vi "Update Reversi Project.vi"() -> ()   [LabVIEW 2020]
uses:
  dev/Version.ctl
  dev/Updater State.ctl
  c5f3ca88-f85c-4b21-a54c-2e2b82621a56.vi
  fab92dee-f5cc-474f-8dc6-a01214f8643b.vi
  <vilib>/Comparison/Equal/Equal Functor/Equal Functor.lvclass
panel:
  out "Project":refnum<vi>
  out "Template Vers Str":string
  out "Project Vers Str":string
  out "Template Version":T1
  out "Project Version":T1
  out "NonOOP Template":path
  out "Progress":u16(slide) scale=0.0..100.0
  out "Status":string
  out "Players":path[](array[path])
  out "OOP Template":path
  out "Engine Folder":path
  out "Project Path":path
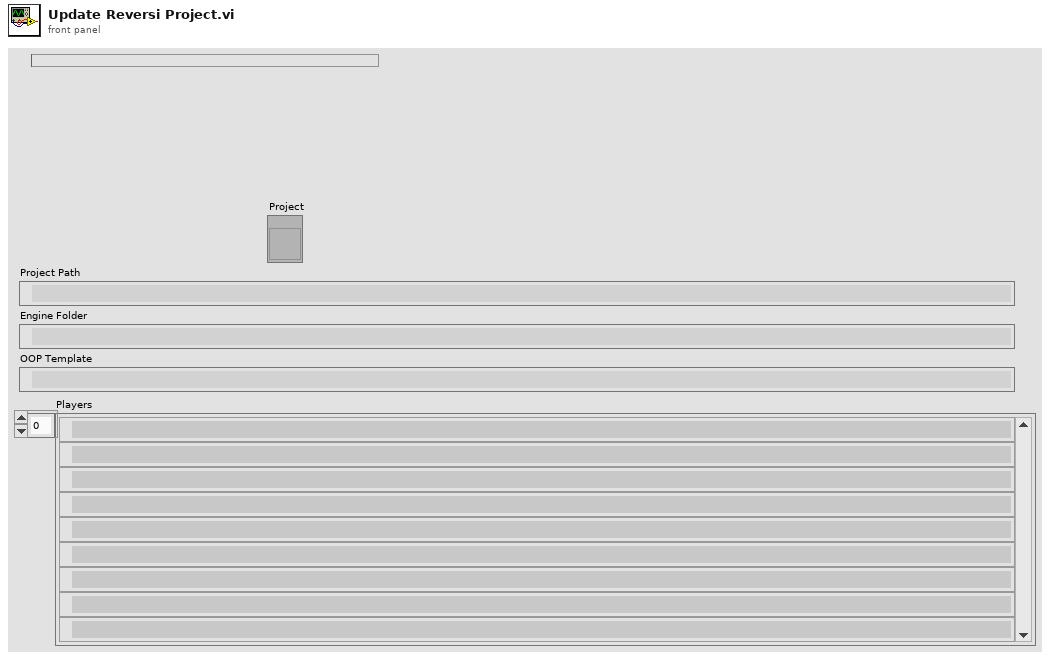
[diagram p1: front panel]
types:
  T1 = typedef "Version.ctl" = cluster{"Major":u16, "Minor":u16, "Fix":u16, "Build":u16}
  T2 = typedef "Updater State.ctl" = enum16{"Get References", "Check Versions", "Confirm", "Close Project", "Copy Engine", "Copy Players", "Open Project", "Version Scripting", "Close"}
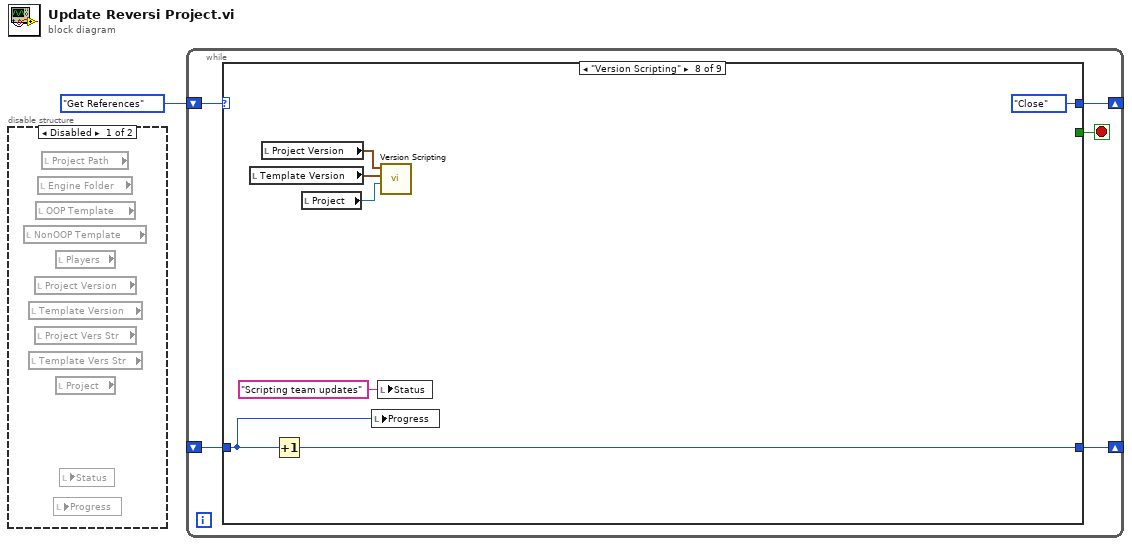
[diagram p0: block diagram]
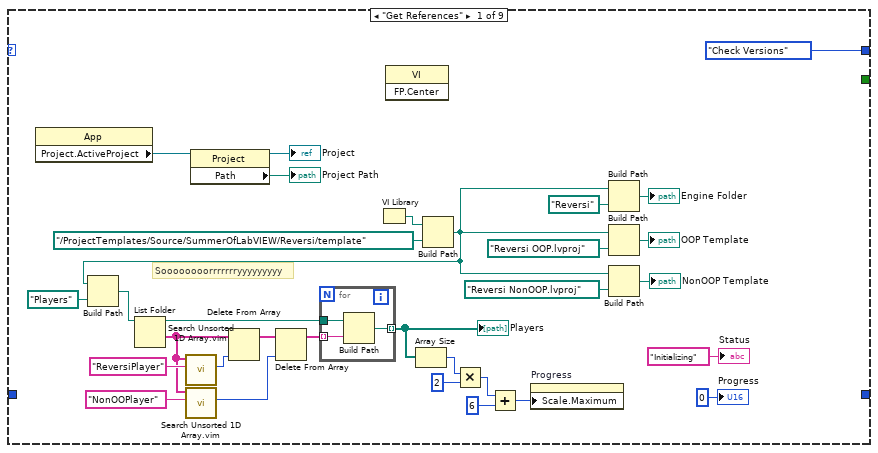
[diagram p3: hidden frame]
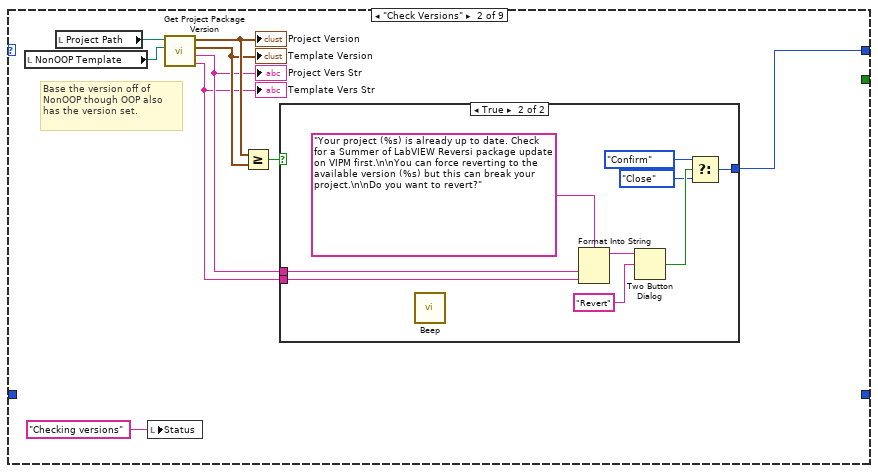
[diagram p4: hidden frame]
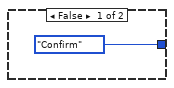
[diagram p5: hidden frame]
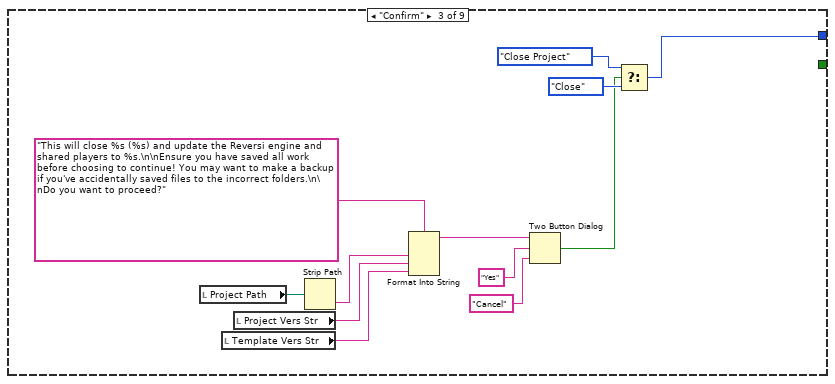
[diagram p6: hidden frame]
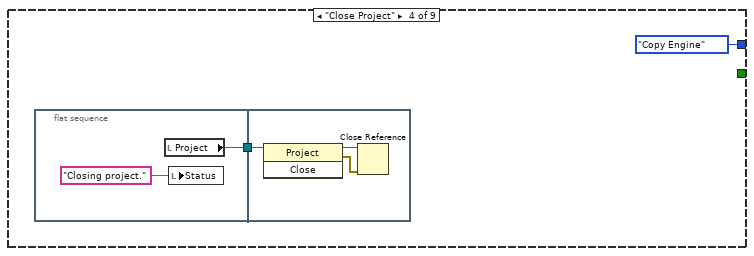
[diagram p7: hidden frame]
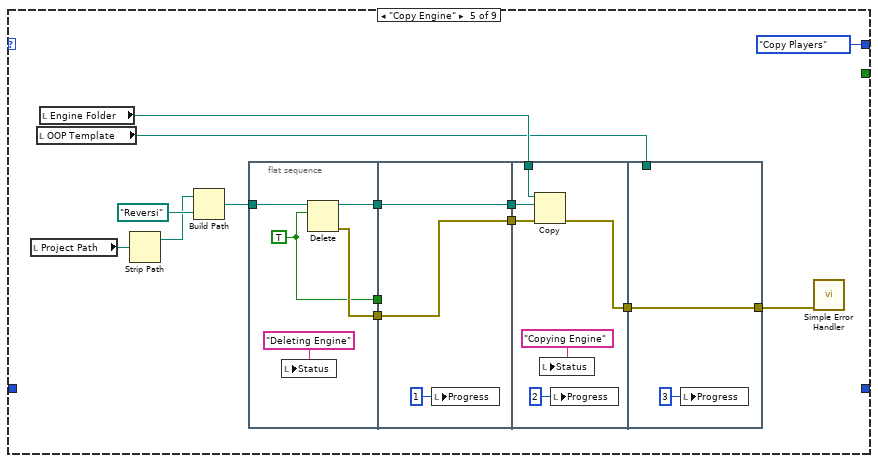
[diagram p8: hidden frame]
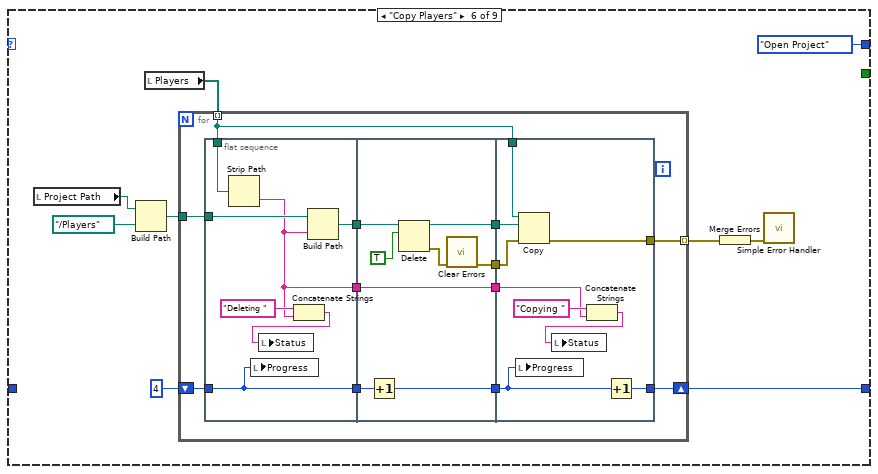
[diagram p9: hidden frame]
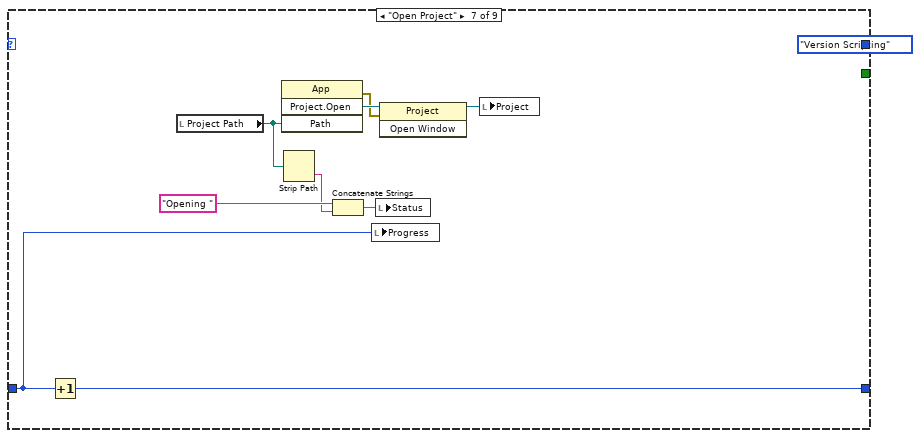
[diagram p10: hidden frame]
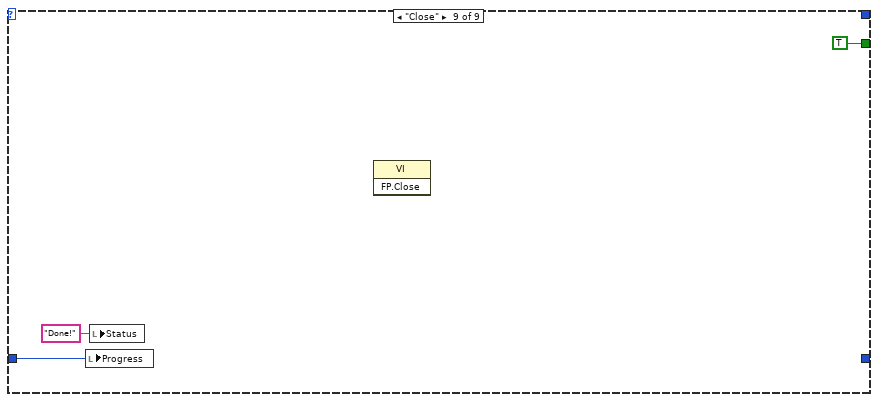
[diagram p11: hidden frame]
diagram:
  n1 = disable-structure shown="Disabled" {
    frame Disabled {
      n2 = local read "NonOOP Template"() -> ()  [unwired: 1 out]
      n3 = local read "Template Version"() -> ()  [unwired: 1 out]
      n4 = local read "Template Vers Str"() -> ()  [unwired: 1 out]
      n5 = local read "Project Version"() -> ()  [unwired: 1 out]
      n6 = local read "Project Vers Str"() -> ()  [unwired: 1 out]
      n7 = local read "OOP Template"() -> ()  [unwired: 1 out]
      n8 = local read "Engine Folder"() -> ()  [unwired: 1 out]
      n9 = local read "Project Path"() -> ()  [unwired: 1 out]
      n10 = local read "Progress"() -> ()  [unwired: 1 in]
      n11 = local read "Players"() -> ()  [unwired: 1 out]
      n12 = local read "Project"() -> ()  [unwired: 1 out]
      n13 = local read "Status"() -> ()  [unwired: 1 in]
    }
    frame Enabled {
    }
  }
  n14 = while {
    shift-right: [w5] -> _
    shift-left: Updater_State."Get References" -> [w6]
    shift-right: [w3] -> _
    shift-left: _ -> [w2]
    stop <- w4 stop-if-true
    n15 = case shown="\"Version Scripting\"" w6 {
      tunnel: [Updater_State."Check Versions" ("f") w43 w66 Updater_State."Copy Engine" ("f") Updater_State."Copy Players" ("f") Updater_State."Open Project" ("f") Updater_State."Version Scripting" ("f") Updater_State."Close" ("f") _] -> w5
      tunnel: [_ _ _ _ _ _ _ _ TRUE] -> w4
      tunnel: [_ _ _ _ _ w109 w155 w164 _] -> w3
      tunnel: w2 -> [_ _ _ _ _ _ w156 w165 w172]
      frame "Get References" {
        # "Soooooooorrrrrrryyyyyyyyy"
        n16 = property class="App"() -> ("Project.ActiveProject"=w15:refnum<vi>)  [unwired: 2 in, 2 out]
        n17 = property class="Project"(reference=w15) -> (reference out=→"Project":refnum<vi>, "Path"=→"Project Path":path)  [unwired: 1 in, 1 out]
        n18 = VI Library() -> (path=w35:path)
        n19 = invoke class="VI" method="FP.Center"() -> ()  [unwired: 3 in, 3 out]
        n20 = Build Path(base path=w35, name or relative path=path "../ProjectTemplates/Source/SummerOfLabVIEW/Reversi/template") -> (appended path=w14:path)
        n21 = Build Path(base path=w14, name or relative path=path "Players") -> (appended path=w28:path)
        n22 = List Folder(path=w28) -> (path out=w25:path, folder names=w10:string[])  [unwired: 3 in, 2 out]
        n23 = call "Search Unsorted 1D Array.vim"("element"="ReversiPlayer", "unsorted 1D array"=w10) -> ("index of element"=w26:i32)  [unwired: 9 in]
        n24 = call "Search Unsorted 1D Array.vim"("element"="NonOOPlayer", "unsorted 1D array"=w10) -> ("index of element"=w8:i32)  [unwired: 9 in]
        n25 = Delete From Array(array=w10, index=w26) -> (array with subset deleted=w9:string[])  [unwired: 1 in, 1 out]
        n26 = Delete From Array(array=w9, index=w8) -> (array with subset deleted=w7:string[])  [unwired: 1 in, 1 out]
        n27 = for {
          tunnel: w7 -> [w39] mode=indexing
          tunnel: w25 -> [w40]
          tunnel: [w38] -> w23 mode=indexing
          n28 = Build Path(base path=w40, name or relative path=w39) -> (appended path=w38:path)
        }
        "Players" <- w23
        n29 = Array Size(array=w23) -> (size(s)=w22:i32)
        n30 = Multiply(x=w22, y=2) -> (x*y=w20:i32)
        n31 = Add(x=w20, y=6) -> (x+y=w18:i32)
        n32 = property on="Progress" class="Slide (strict)"("Scale.Maximum"=w18) -> ()  [unwired: 2 in, 2 out]
        n33 = Build Path(base path=w14, name or relative path=path "Reversi") -> (appended path=→"Engine Folder":path)
        n34 = Build Path(base path=w14, name or relative path=path "Reversi OOP.lvproj") -> (appended path=→"OOP Template":path)
        n35 = Build Path(base path=w14, name or relative path=path "Reversi NonOOP.lvproj") -> (appended path=→"NonOOP Template":path)
        "Status" <- "Initializing" ("Status")
        "Progress" <- u16 0 ("Progress")
      }
      frame "Check Versions" {
        # "Base the version off of NonOOP though OOP also has the version set."
        n36 = local read "NonOOP Template"() -> (w47:path)
        n37 = local read "Project Path"() -> (w49:path)
        n38 = local write "Status"("Checking versions" ("Status")) -> ()
        n39 = call "Get Project Package Version.vi"("Template Project"=w47, "Project Path"=w49) -> ("Template Vers Str"=w41:string, "Project Vers Str"=w42:string, "Template Version"=w45:T1, "Project Version"=w46:T1)  [unwired: 6 in]
        "Project Version" <- w46
        "Template Version" <- w45
        "Project Vers Str" <- w42
        "Template Vers Str" <- w41
        n40 = Greater Or Equal?(x=w46, y=w45) -> (x >= y?=w44:bool)
        n41 = case shown="True" w44 {
          tunnel: [Updater_State."Confirm" ("f") w51] -> w43
          tunnel: w42 -> [_ w58]
          tunnel: w41 -> [_ w57]
          frame False {
          }
          frame True {
            n42 = call <vilib>:"Beep.vi"() -> ()  [unwired: 12 in]
            n43 = Format Into String(format string="Your project (%s) is already up to date. Check for a Summer of LabVIEW Reversi package update on VIPM first.\n\nYou can force reverting to the available version (%s) but this can break your project.\n\nDo you want to revert?" ("message"), w58, w57) -> (resulting string=w56:string)  [unwired: 2 in, 1 out]
            n44 = Two Button Dialog(message=w56, 2:"Revert" ("T button name (\"OK\")")) -> (T button?=w54:bool)  [unwired: 1 in]
            n45 = Select(t=Updater_State."Confirm" ("f"), s=w54, f=Updater_State."Close") -> (s? t:f=w51:T2)
          }
        }
      }
      frame "Confirm" {
        n46 = local read "Project Path"() -> (w64:path)
        n47 = local read "Template Vers Str"() -> (w60:string)
        n48 = local read "Project Vers Str"() -> (w61:string)
        n49 = Strip Path(path=w64) -> (name=w63:string)  [unwired: 1 out]
        n50 = Format Into String(format string="This will close %s (%s) and update the Reversi engine and shared players to %s.\n\nEnsure you have saved all work before choosing to continue! You may want to make a backup if you've accidentally saved files to the incorrect folders.\n\nDo you want to proceed?" ("message"), w63, w61, w60) -> (resulting string=w62:string)  [unwired: 2 in, 1 out]
        n51 = Two Button Dialog(message=w62, 1:"Cancel" ("F button name (\"Cancel\")"), 2:"Yes" ("T button name (\"OK\")")) -> (T button?=w67:bool)
        n52 = Select(t=Updater_State."Close Project", s=w67, f=Updater_State."Close") -> (s? t:f=w66:T2)
      }
      frame "Close Project" {
        n53 = flat-sequence {
          tunnel: [w74] -> w72
          tunnel: w72 -> [w76]
          frame #0 {
            n54 = local read "Project"() -> (w74:refnum<vi>)
            n55 = local write "Status"("Closing project." ("Status")) -> ()
          }
          frame #1 {
            n56 = invoke class="Project" method="Close"(reference=w76) -> (reference out=w78:refnum<vi>, error out=w77:errorcluster)  [unwired: 2 in, 1 out]
            n57 = Close Reference(reference=w78, error in (no error)=w77) -> ()  [unwired: 1 out]
          }
        }
      }
      frame "Copy Engine" {
        n58 = local read "Project Path"() -> (w92:path)
        n59 = local read "OOP Template"() -> (w80:path)
        n60 = local read "Engine Folder"() -> (w82:path)
        n61 = Strip Path(path=w92) -> (stripped path=w90:path)  [unwired: 1 out]
        n62 = Build Path(base path=w90, name or relative path=path "Reversi") -> (appended path=w89:path)
        n63 = flat-sequence {
          tunnel: w89 -> [w96]
          tunnel: [w97] -> w87
          tunnel: [w95] -> w86
          tunnel: [w94] -> w85
          tunnel: w87 -> [w98]
          tunnel: w86 -> [w100]
          tunnel: w85 -> [_]
          tunnel: [w100] -> w84
          tunnel: [w98] -> w83
          tunnel: w84 -> [w105]
          tunnel: w83 -> [w106]
          tunnel: w82 -> [w104]
          tunnel: [w103] -> w81
          tunnel: w81 -> [w107]
          tunnel: w80 -> [_]
          tunnel: [w107] -> w79
          frame #0 {
            w94 = TRUE ("entire hierarchy (F)")
            n64 = local write "Status"("Deleting Engine") -> ()
            n65 = Delete(path (use dialog)=w96, entire hierarchy (F)=w94) -> (deleted path=w95:path, error out=w97:errorcluster)  [unwired: 3 in, 1 out]
          }
          frame #1 {
            n66 = local write "Progress"(u16 1 ("Progress")) -> ()
          }
          frame #2 {
            n67 = Copy(8:w106, 10:w105, 11:w104) -> (0:w103:errorcluster)  [unwired: 2 in, 2 out]
            n68 = local write "Status"("Copying Engine") -> ()
            n69 = local write "Progress"(u16 2 ("Progress")) -> ()
          }
          frame #3 {
            n70 = local write "Progress"(u16 3 ("Progress")) -> ()
          }
        }
        n71 = call <vilib>:"Simple Error Handler.vi"("error in (no error)"=w79) -> ()  [unwired: 4 in, 5 out]
      }
      frame "Copy Players" {
        n72 = local read "Project Path"() -> (w117:path)
        n73 = Build Path(base path=w117, name or relative path=path "../Players") -> (appended path=w114:path)
        n74 = local read "Players"() -> (w115:path[])
        n75 = for {
          tunnel: w115 -> [w125] mode=indexing
          tunnel: w114 -> [w129]
          tunnel: [w124] -> w113 mode=indexing
          shift-right: [w118] -> w109
          shift-left: u16 4 ("Progress") -> [w121]
          n76 = flat-sequence {
            tunnel: w129 -> [w136]
            tunnel: w125 -> [w134]
            tunnel: [w135] -> w128
            tunnel: [w131] -> w122
            tunnel: w121 -> [w130]
            tunnel: [w130] -> w120
            tunnel: w128 -> [w142]
            tunnel: [w141] -> w127
            tunnel: [w140] -> w126
            tunnel: [w139] -> w123
            tunnel: w122 -> [w139]
            tunnel: w120 -> [w138]
            tunnel: [w137] -> w119
            tunnel: w127 -> [w153]
            tunnel: w126 -> [w152]
            tunnel: w125 -> [w151]
            tunnel: [w150] -> w124
            tunnel: w123 -> [w145]
            tunnel: w119 -> [w149]
            tunnel: [w148] -> w118
            frame #0 {
              n77 = Strip Path(path=w134) -> (name=w131:string)  [unwired: 1 out]
              n78 = local write "Progress"(w130) -> ()
              n79 = Concatenate Strings("Deleting ", w131) -> (w132:string)
              n80 = local write "Status"(w132) -> ()
              n81 = Build Path(base path=w136, name or relative path=w131) -> (appended path=w135:path)
            }
            frame #1 {
              n82 = Increment(x=w138) -> (x+1=w137:u16)
              n83 = Delete(path (use dialog)=w142, entire hierarchy (F)=TRUE) -> (deleted path=w140:path, error out=w144:errorcluster)  [unwired: 3 in, 1 out]
              n84 = call <vilib>:"Clear Errors.vi"("error in (no error)"=w144) -> ("error out"=w141:errorcluster)  [unwired: 5 in, 1 out]
            }
            frame #2 {
              n85 = local write "Progress"(w149) -> ()
              n86 = Copy(8:w153, 10:w152, 11:w151) -> (0:w150:errorcluster)  [unwired: 2 in, 2 out]
              n87 = Concatenate Strings("Copying ", w145) -> (w147:string)
              n88 = local write "Status"(w147) -> ()
              n89 = Increment(x=w149) -> (x+1=w148:u16)
            }
          }
        }
        n90 = Merge Errors(w113) -> (w112:errorcluster)
        n91 = call <vilib>:"Simple Error Handler.vi"("error in (no error)"=w112) -> ()  [unwired: 4 in, 5 out]
      }
      frame "Open Project" {
        n92 = Increment(x=w156) -> (x+1=w155:u16)
        n93 = local read "Project Path"() -> (w160:path)
        n94 = invoke class="App" method="Project.Open"("Path"=w160) -> (error out=w161:errorcluster, "Project:Open"=w162:refnum<vi>)  [unwired: 3 in, 2 out]
        n95 = Strip Path(path=w160) -> (name=w158:string)  [unwired: 1 out]
        n96 = Concatenate Strings("Opening " ("Status"), w158) -> (w157:string)
        n97 = local write "Progress"(w156) -> ()
        n98 = local write "Status"(w157) -> ()
        n99 = invoke class="Project" method="Open Window"(reference=w162, error in=w161) -> (reference out=w154:refnum<vi>)  [unwired: 1 in, 2 out]
        n100 = local write "Project"(w154) -> ()
      }
      frame "Version Scripting" {
        n101 = local read "Template Version"() -> (w170:T1)
        n102 = local read "Project Version"() -> (w169:T1)
        n103 = Increment(x=w165) -> (x+1=w164:u16)
        n104 = local read "Project"() -> (w168:refnum<vi>)
        n105 = local write "Progress"(w165) -> ()
        n106 = local write "Status"("Scripting team updates" ("Status")) -> ()
        n107 = call "Version Scripting.vi"("Project"=w168, "To"=w170, "From"=w169) -> ()  [unwired: 9 in]
      }
      frame "Close" {
        n108 = local write "Progress"(w172) -> ()
        n109 = local write "Status"("Done!" ("Status")) -> ()
        n110 = invoke class="VI" method="FP.Close"() -> ()  [unwired: 3 in, 3 out]
      }
    }
  }
